vi "Bertta_v08_51.vi"() -> ()   [LabVIEW 2015]
panel:
  out "Started:":string
  in  "SHUTDOWN":bool
  in  "MASTER CONTROL":bool
  in  "Tab Control":T1(tab)
  in  "Read Seq":bool
  in  "Save Seq":bool
  in  "Configuration file":path=path "C:/Users/shresplab/Desktop/BerttaConfiguration.lvm" caption="Filename"
  in  "OK Button 2":bool
  out "Boolean":bool
  in  "User (initials)":string
  in  "Project name":string
  in  "Description":string
  out "Output file":string
  out "Sensor OK 6":bool
  out "Sensor OK 5":bool
  out "Sensor OK 4":bool
  out "Sensor OK 3":bool
  in  "OK Button":bool
  in  "Add comment":string
  out "PUMP 1":bool
  out "Target amount":dbl
  out "Scale weight":dbl
  out "Amount now":dbl
  out "Flow rate":dbl
  out "Time to target":dbl format="%<%H:%M:%S>t"
  out "Current step":dbl
  out "Target amount":dbl
  out "Amount now":dbl
  out "Tr":dbl
  out "Tj in":dbl
  out "Tj out":dbl
  out "T set":dbl
  out "Current step":i32
  out "RPM":dbl
  out "Torque 2":dbl
  out "Waveform Chart 5":dynamicdata(graph)
  out "Waveform Chart 6":dynamicdata(graph)
  out "Waveform Chart 7":dynamicdata(graph)
  out "Amount now":dbl
  out "Target amount":dbl
  out "Current step":dbl
  out "Time to target":dbl format="%<%H:%M:%S>t"
  out "Flow rate":dbl
  out "Amount now":dbl
  out "Scale weight":dbl
  out "Target amount":dbl
  out "PUMP 2":bool
  in  "Tab Control 2":T2(tab)
  out "Waveform Chart 3":dynamicdata(graph)
  out "Waveform Chart 8":dynamicdata(graph)
  out "Waveform Chart 11":dynamicdata(graph)
  out "Waveform Chart 9":dynamicdata(graph)
  out "Table":string[][](table)=[["14.8.2017 18.06.59", "0,000000", "417,670000", "-0,150000", "1,000000", "22,220000", "23,366837", "23,574959", "23,985852", "23,690000", "240,000000", "4,000000", "0,000000", "397,000000", "-397,000000", "1,000000"], ["14.8.2017 18.07.06", "0,000000", "417,640000", "-0,120000", "1,000000", "22,220000", "23,763115", "23,906257", "23,985694", "23,680000", "240,000000", "4,000000", "0,000000", "397,000000", "-397,000000", "1,000000"], ["14.8.2017 18.07.13", "0,000000", "417,640000", "-0,120000", "1,000000", "22,220000", "23,965922", "24,013440", "23,984906", "23,670000", "240,000000", "4,100000", "3,000000", "397,000000", "-397,000000", "1,000000"], ["14.8.2017 18.07.21", "0,000000", "417,640000", "-0,120000", "1,000000", "22,220000", "23,943860", "23,900110", "23,987113", "23,670000", "240,000000", "4,000000", "0,000000", "397,000000", "-397,000000", "1,000000"], ["14.8.2017 18.07.28", "0,000000", "417,640000", "-0,120000", "1,000000", "22,220000", "23,736328", "23,600018", "23,989004", "23,660000", "240,000000", "4,000000", "0,000000", "397,000000", "-397,000000", "1,000000"], ["14.8.2017 18.07.36", "0,000000", "417,640000", "-0,120000", "1,000000", "22,220000", "23,480910", "23,324538", "23,991053", "23,660000", "240,000000", "4,000000", "0,000000", "397,000000", "-397,000000", "1,000000"], ["14.8.2017 18.07.43", "0,000000", "417,640000", "-0,120000", "2,000000", "22,220000", "23,195579", "23,008270", "23,999093", "23,650000", "240,000000", "4,000000", "0,000000", "397,000000", "-397,000000", "1,000000"], ["14.8.2017 18.07.51", "0,000000", "417,650000", "-417,650000", "1,000000", "22,220000", "22,862541", "22,649021", "24,003979", "23,650000", "240,000000", "4,000000", "0,000000", "397,000000", "-397,000000", "2,000000"], ["14.8.2017 18.07.58", "0,000000", "417,640000", "0,010000", "1,000000", "22,220000", "22,541353", "22,354878", "24,005398", "23,650000", "240,000000", "4,000000", "0,000000", "397,000000", "-397,000000", "1,000000"], ["14.8.2017 18.08.06", "0,000000", "417,640000", "0,010000", "1,000000", "22,220000", "22,347931", "22,253738", "24,007605", "23,640000", "240,000000", "4,100000", "0,000000", "397,000000", "-397,000000", "1,000000"], ["14.8.2017 18.08.13", "0,000000", "417,640000", "0,010000", "1,000000", "22,220000", "22,329030", "22,302102", "24,006028", "23,640000", "240,000000", "4,000000", "0,000000", "395,820000", "-395,820000", "1,000000"], ["14.8.2017 18.08.20", "0,000000", "417,640000", "0,010000", "1,000000", "22,220000", "22,466849", "22,511320", "24,002403", "23,630000", "240,000000", "4,000000", "0,000000", "395,830000", "-0,010000", "1,000000"], ["14.8.2017 18.08.28", "0,000000", "417,640000", "0,010000", "1,000000", "22,220000", "22,707062", "22,835101", "24,000984", "23,620000", "240,000000", "4,000000", "0,000000", "395,830000", "-0,010000", "1,000000"], ["14.8.2017 18.08.35", "0,000000", "417,640000", "0,010000", "1,000000", "22,220000", "23,054104", "23,232979", "24,001299", "23,600000", "240,000000", "4,000000", "0,000000", "395,830000", "-0,010000", "1,000000"], ["14.8.2017 18.08.43", "0,000000", "417,640000", "0,010000", "1,000000", "22,220000", "23,412371", "23,522793", "24,002560", "23,590000", "240,000000", "4,000000", "0,000000", "395,820000", "0,000000", "1,000000"], ["14.8.2017 18.08.51", "0,000000", "417,640000", "0,010000", "1,000000", "22,220000", "23,596247", "23,656125", "24,003821", "23,580000", "240,000000", "4,000000", "0,000000", "395,820000", "0,000000", "1,000000"]]
  in  "T ext / T ext 2":enum32{"External 1", "External 2"}(radio)
  out "Sensor OK":bool
  in  "T fail":dbl=20.0
  out "Boolean 12":bool
  out "Boolean 7":bool
  out "Boolean 6":bool
  out "Boolean 5":bool
  out "Boolean 4":bool
  in  "?":bool
  in  "T setpoint":dbl=20.0
  in  "Lauda port":dbl=9.0
  out "Data out":dbl
  in  "Bypass select":enum32{"Tr", "Tj"}(radio)
  in  "TempSeq":dbl[][](array[numeric])=[[20.0, 45.0, 50.0, 46.0], [46.0, 50.0, 20.0, 51.0], [20.0, 50.0, 3.0, 25.0], [20.0, 20.0, 0.0, 20.0], [20.0, 20.0, 0.0, 20.0], [20.0, 20.0, 1000.0, 20.0]]
  out "T control":dbl
  out "Tr":dbl
  out "Tj in":dbl
  out "Tj out":dbl
  out "DT":dbl
  out "Elapsed":i32
  in  "PAUSE":bool
  out "Boolean 19":bool
  in  "Reset":bool
  in  "Treshold (Tset)":dbl=1.0
  in  "Tmax":dbl=199.0
  in  "Tmin":dbl=20.0
  out "Current step":i32
  out "Tset":dbl
  out "Waveform Chart":dynamicdata(graph)
  out "T external 2":dbl
  in  "Xe":dbl=1.0
  in  "Ring":u16(ring) items=["SCALE 1", "SCALE 2", "SCALE 3"]
  out "Data out":dbl
  out "Port":i32=10
  in  "Radio Buttons":enum32{"Reglo Digital", "Reglo Analog", "PAM"}(radio)=enum."Reglo Analog"
  out "Speed":dbl
  out "mA":dbl format="%#_2g"
  in  "Port":i32=16
  out "RPM":dbl format="%#_2g"
  out "Boolean 18":bool
  out "Boolean 17":bool
  out "Boolean 16":bool
  out "Boolean 15":bool
  out "Boolean 14":bool
  out "Boolean 13":bool
  out "Boolean 11":bool
  out "Boolean 10":bool
  out "Boolean 9":bool
  out "Boolean 8":bool
  in  "PumpSeq":dbl[][](array[numeric])=[[3.0, 3.0, 7.0], [2.0, 2.0, 2.0], [4.0, 2.0, 100.0], [0.0, 0.0, 0.0], [0.0, 0.0, 0.0], [0.0, 0.0, 0.0], [0.0, 0.0, 0.0], [0.0, 0.0, 0.0], [0.0, 0.0, 0.0], [0.0, 0.0, 0.0], [0.0, 1.0, 0.0]]
  in  "?":bool
  out "Flow rate (g/min)":dbl
  out "Time (min)":dbl
  out "Target (g)":dbl
  out "Scale reading":dbl
  out "Step amount now":dbl
  out "Time to target":dbl format="%<%H:%M:%S>t"
  in  "Grams / min":dbl
  out "Waveform Chart 2":dynamicdata(graph)
  in  "?":bool
  out "Total amount now":dbl
  out "Total time":dbl
  out "Total amount target":dbl
  out "Boolean 20":bool
  in  "Reset 2":bool
  out "Waveform Chart 10":dynamicdata(graph)
  in  "Reset 3":bool
  out "Boolean 31":bool
  out "Total amount target 2":dbl
  out "Total time 2":dbl
  out "Boolean 30":bool
  out "Boolean 29":bool
  out "Boolean 28":bool
  out "Boolean 27":bool
  out "Boolean 26":bool
  out "Boolean 25":bool
  out "Boolean 24":bool
  out "Boolean 23":bool
  out "Boolean 22":bool
  out "Boolean 21":bool
  in  "PumpSeq 2":dbl[][](array[numeric])=[[3.0, 3.0, 7.0], [2.0, 2.0, 2.0], [4.0, 2.0, 100.0], [0.0, 0.0, 0.0], [0.0, 0.0, 0.0], [0.0, 0.0, 0.0], [0.0, 0.0, 0.0], [0.0, 0.0, 0.0], [0.0, 0.0, 0.0], [0.0, 0.0, 0.0], [0.0, 1.0, 0.0]]
  in  "Ring 2":u16(ring)=1 items=["SCALE 1", "SCALE 2", "SCALE 3"]
  out "Data out 2":dbl
  out "Port 3":i32=10
  in  "Radio Buttons 2":enum32{"Reglo Digital", "Reglo Analog", "PAM"}(radio)
  out "RPM":dbl format="%#_2g"
  in  "Port":i32=15
  out "mA":dbl format="%#_2g"
  out "Speed":dbl
  in  "?":bool
  in  "Grams / min":dbl
  out "Time (min)":dbl
  out "Target (g)":dbl
  out "Total amount now":dbl
  out "Time to target":dbl format="%<%H:%M:%S>t"
  in  "?":bool
  out "Step amount now":dbl
  out "Scale reading":dbl
  out "Flow rate (g/min)":dbl
  in  "Bypass select 2":enum32{"Remote", "Manual"}(radio)
  in  "Port":dbl=13.0
  out "RPM":dbl
  out "Torque":dbl
  in  "Set RPM":dbl(slide) scale=0.0..500.0
  out "Waveform Chart 4":dynamicdata(graph)
  out "DAQ 9217 (PT100)":errorcluster
  # "PUMP & SCALE 1"
  # "PUMP & SCALE 2"
  # "STEP"
  # "STEP"
  # "TOTAL"
  # "TOTAL"
  # "Temperature sensor:"
  # "Manual control:"
  # "Tinit     >    Tset       Min. time      Tfail"
  # "Manual control / end of sequence"
  # "Manual control"
  # "Secondary temperature sensor"
  # "Device communication"
  # "Grams    /   min"
  # "End of sequence"
  # "Manual control"
  # "Device communication"
  # "Pump configuration"
  # "Scale configuration"
  # "Grams    /   min"
  # "End of sequence"
  # "Manual control"
  # "Device communication"
  # "Pump configuration"
  # "Scale configuration"
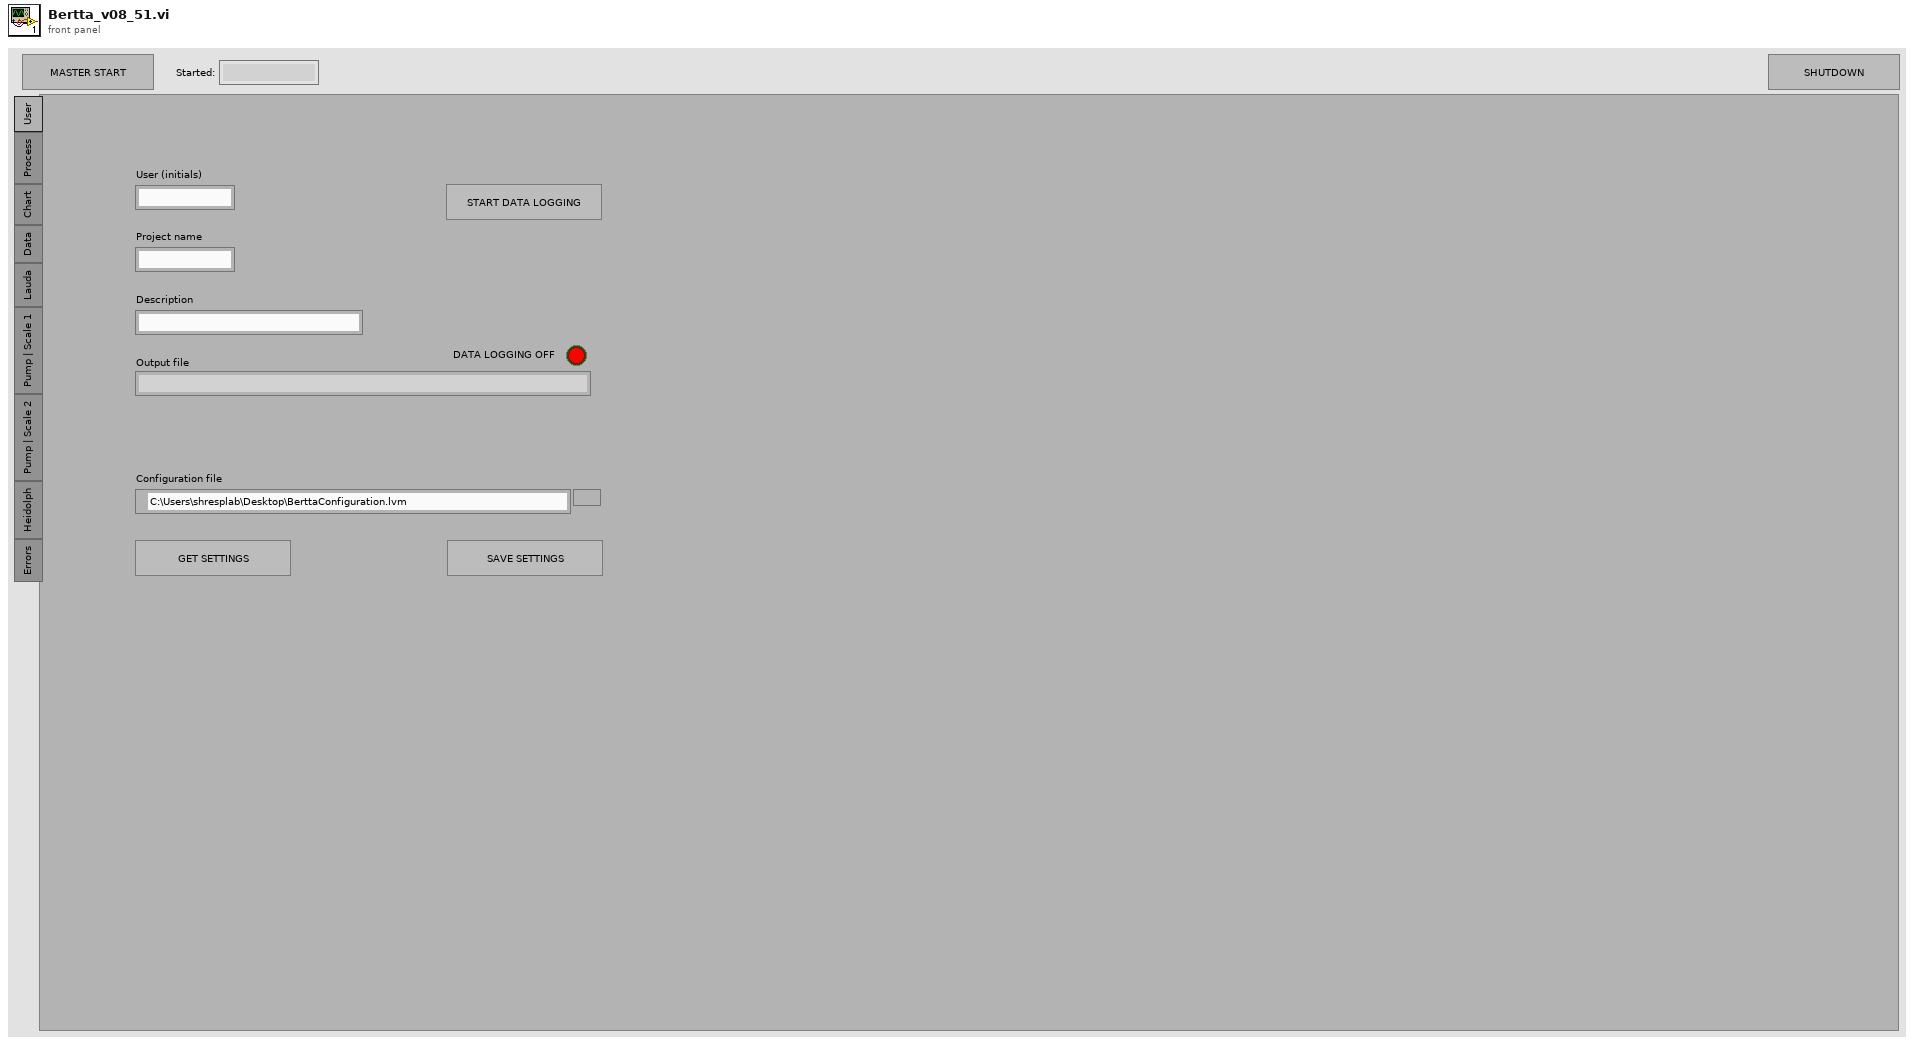
[diagram p1: front panel]
types:
  T1 = enum32{"User", "Process", "Chart", "Data", "Lauda", "Pump | Scale 1", "Pump | Scale 2", "Heidolph", "Errors"}
  T2 = enum32{"Temperatures", "Scale / Pump 1", "Scale / Pump 2", "RPM / torque"}
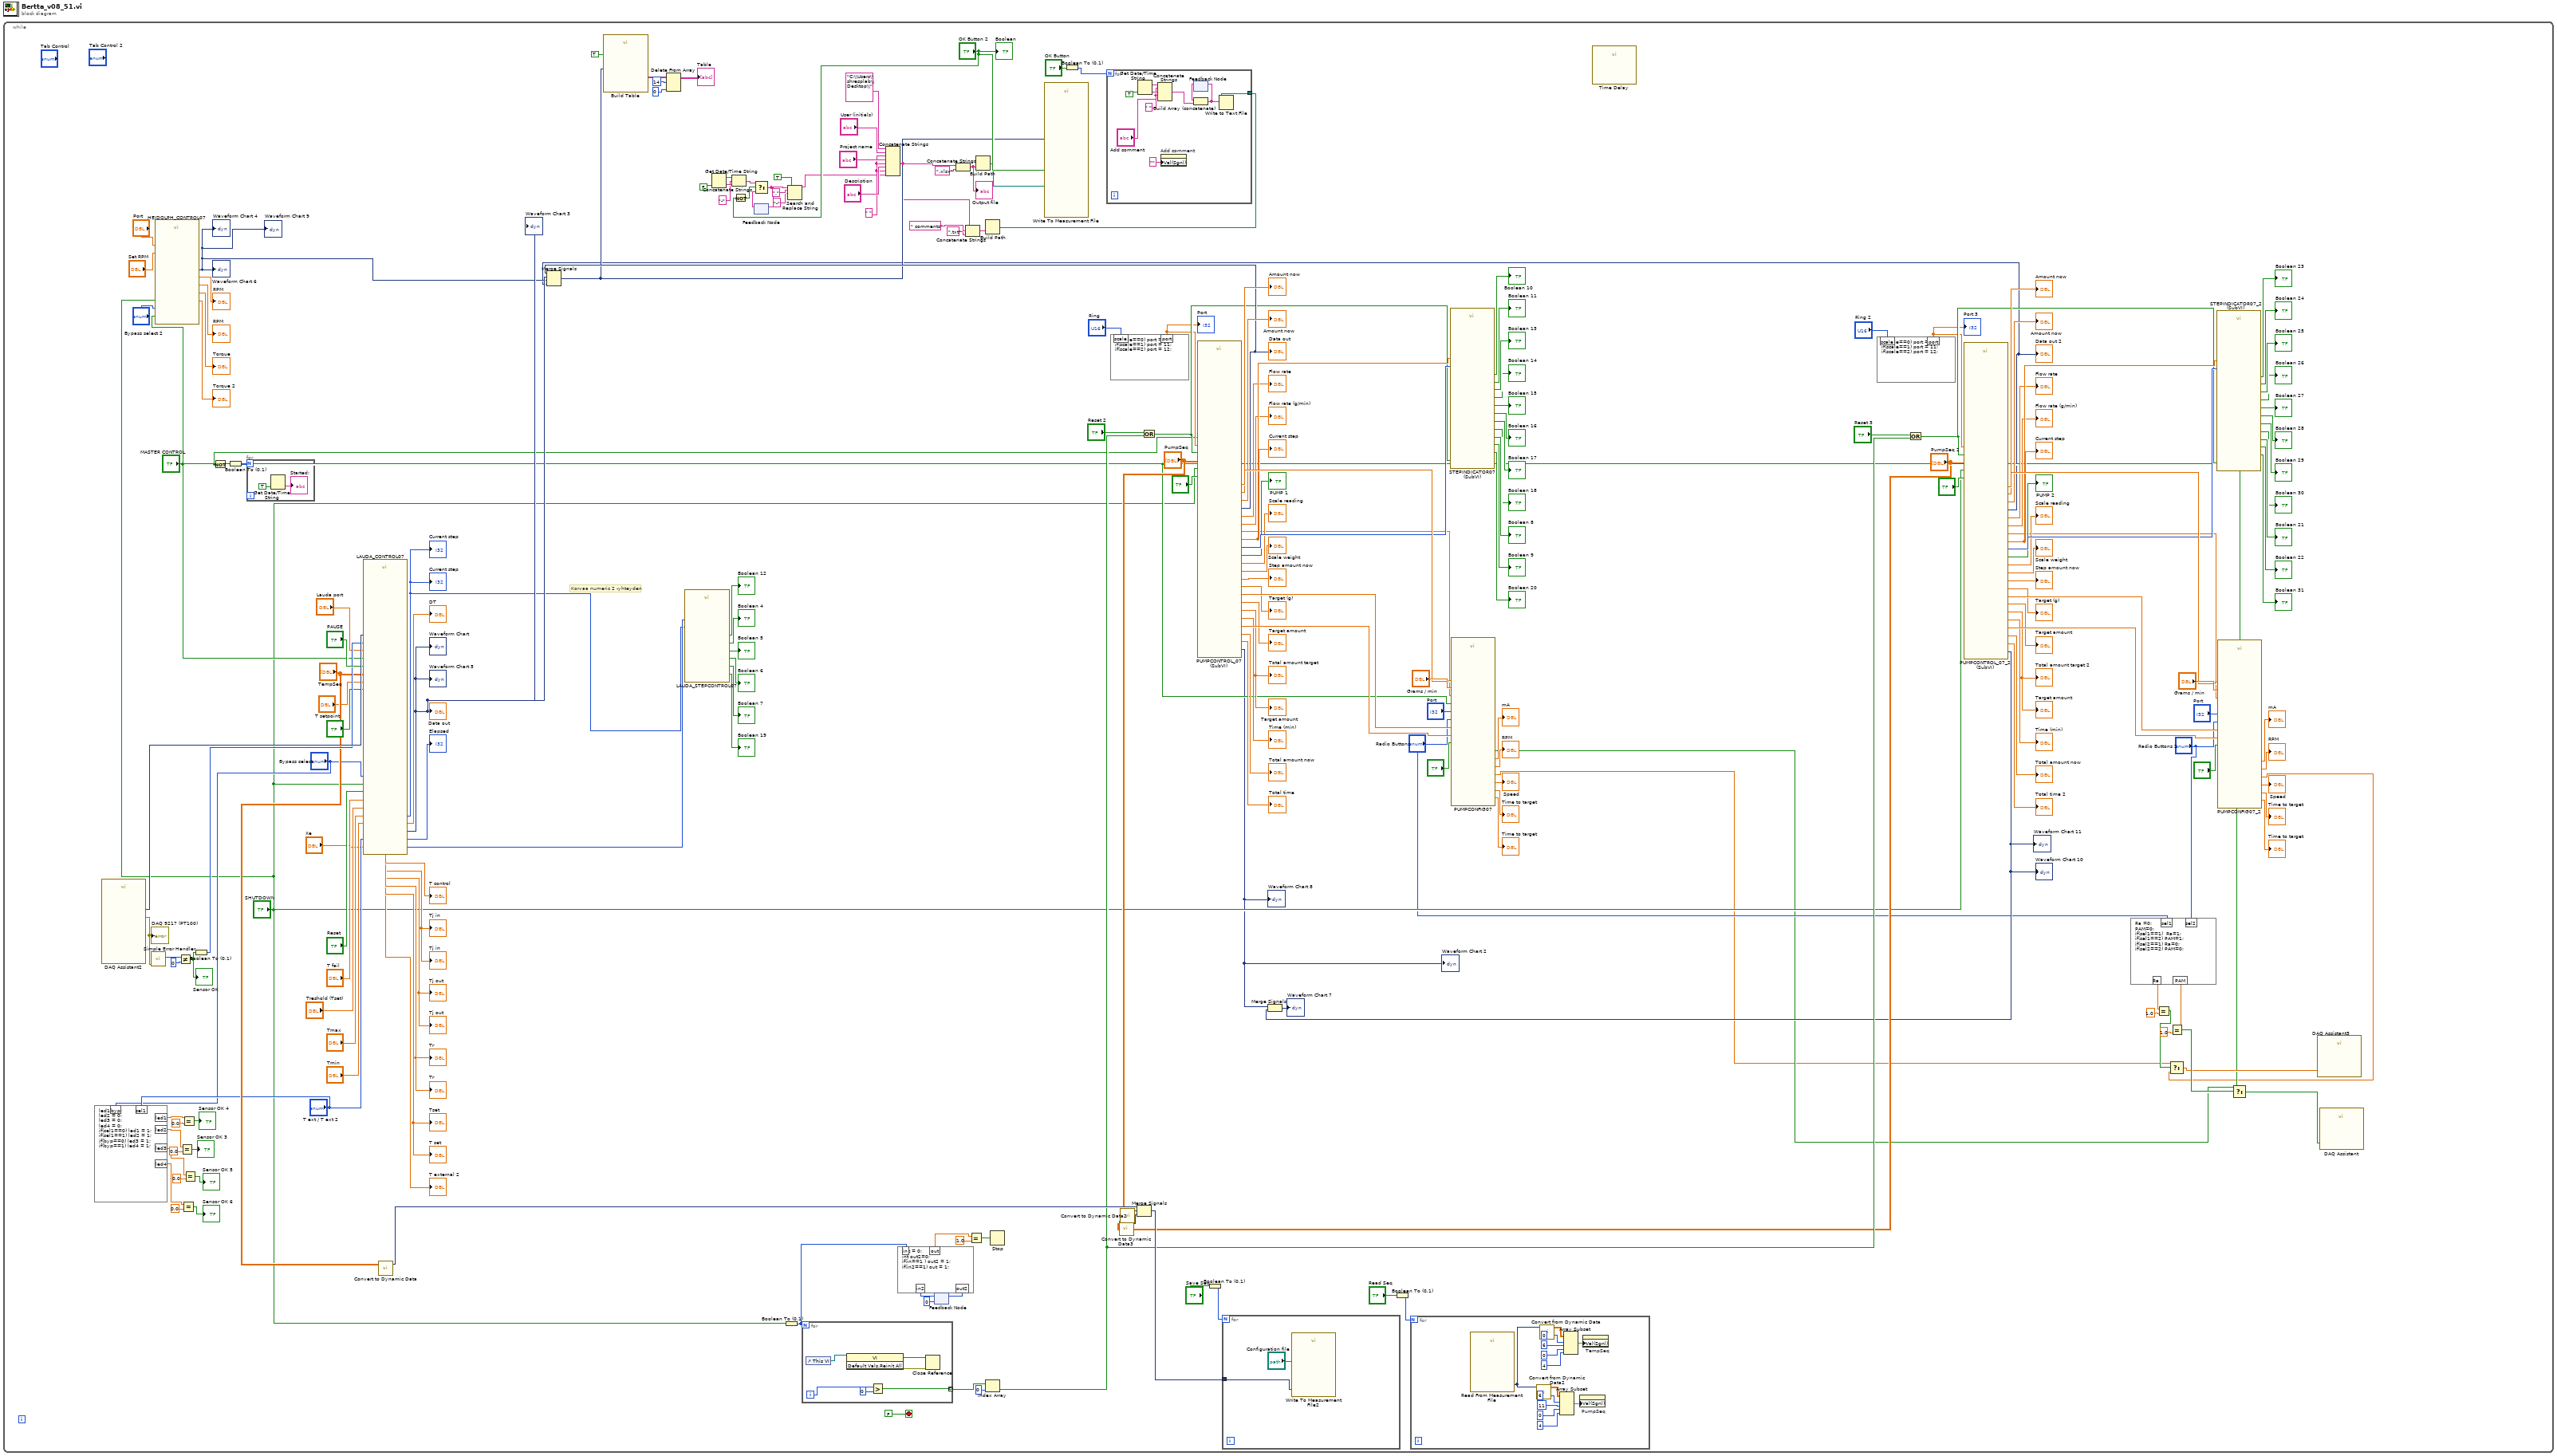
[diagram p0: block diagram]
diagram:
  n1 = while {
    stop <- FALSE stop-if-true
    w157 = " "
    # "Korvaa numeric 2 -yhteyden"
    n2 = formula code="led1 = 0;\nled2 = 0;\nled3 = 0;\nled4 = 0;\nif(sel1==0) led1 = 1;\nif(sel1==1) led2 = 1;\nif(byp==0) led3 = 1;\nif(byp==1) led4 = 1;"("sel1"="T ext / T ext 2", "byp"="Bypass select") -> ("led1"=w81:dbl, "led2"=w79:dbl, "led3"=w74:dbl, "led4"=w73:dbl)
    n3 = call "DAQ Assistant2"() -> ("data"=w220:dynamicdata, "error out"=w164:errorcluster)  [unwired: 17 in, 1 out]
    "DAQ 9217 (PT100)" <- w164
    n4 = call <vilib>:"Simple Error Handler.vi"("error in (no error)"=w164) -> ("code out"=w163:i32)  [unwired: 4 in, 4 out]
    n5 = call "HEIDOLPH_CONTROL07.vi"("master"="MASTER CONTROL", "shutdown"="SHUTDOWN", "Bypass select"="Bypass select 2", "Set RPM"="Set RPM", "Device port"="Port") -> ("Dynamic Data"=w169:dynamicdata, "RPM"=→"RPM":dbl, "RPM 2"=→"RPM":dbl, "Torque"=→"Torque":dbl, "Torque 2"=→"Torque 2":dbl)  [unwired: 2 in]
    "Waveform Chart 4" <- w169
    "Waveform Chart 6" <- w169
    "Waveform Chart 9" <- w169
    n6 = Not Equal?(x=w163, y=0) -> (x != y?=w129:bool)
    "Sensor OK" <- w129
    n7 = Equal?(x=w79, y=0.0) -> (x = y?=→"Sensor OK 3":bool)
    n8 = Equal?(x=w73, y=0.0) -> (x = y?=→"Sensor OK 6":bool)
    n9 = Equal?(x=w81, y=0.0) -> (x = y?=→"Sensor OK 4":bool)
    n10 = Equal?(x=w74, y=0.0) -> (x = y?=→"Sensor OK 5":bool)
    n11 = Boolean To (0,1)(Boolean=w129) -> (0, 1=w161:i16)
    n12 = Not(x="MASTER CONTROL") -> (.not. x?=w146:bool)
    n13 = Boolean To (0,1)(Boolean=w146) -> (0, 1=w147:i16)
    n14 = for {
      N: w147 -> [_]
      n15 = Get Date/Time String(want seconds? (F)=TRUE) -> (time string=→"Started:":string)  [unwired: 2 in, 1 out]
    }
    n16 = call "LAUDA_CONTROL07.vi"("Bypass"="?", "PAUSE"="PAUSE", "data"=w220, "Seq"="TempSeq", "Lauda port"="Lauda port", "Tbypass"="T setpoint", "Treshold"="Treshold (Tset)", "Bypass select"="Bypass select", "err"=w161, "Shutdown"="SHUTDOWN", "Master Start"="MASTER CONTROL", "Reset"="Reset", "Tfail (manual)"="T fail", "Tmax"="Tmax", "Xe"="Xe", "T ext / T ext 2"="T ext / T ext 2", "Tmin"="Tmin") -> ("Tj in"=→"Tj in" →"Tj in":dbl, "DT"=→"DT":dbl, "Tj out"=→"Tj out" →"Tj out":dbl, "Tset"=→"Tset" →"T set":dbl, "Dynamic Data"=w171:dynamicdata, "T ext 2"=→"T external 2":dbl, "Numeric"=w150:i16, "T control"=→"T control":dbl, "Current step"=w2:i32, "Elapsed"=→"Elapsed":i32, "Tr"=→"Tr" →"Tr":dbl)
    "Waveform Chart 3" <- w171
    "Waveform Chart" <- w171
    "Current step" <- w2
    "Data out" <- w171
    "Waveform Chart 5" <- w171
    "Current step" <- w2
    n17 = call "Convert to Dynamic Data"("2D Array"="TempSeq") -> ("Dynamic Data Type"=w139:dynamicdata)  [unwired: 3 in]
    n18 = call "LAUDA_STEPCONTROL07.vi"("Numeric 2"=w2, "Numeric"=w150) -> ("Boolean 13"=→"Boolean 19":bool, "Boolean 6"=→"Boolean 6":bool, "Boolean 5"=→"Boolean 5":bool, "Boolean 4"=→"Boolean 4":bool, "Boolean 7"=→"Boolean 7":bool, "Boolean 12"=→"Boolean 12":bool)  [unwired: 4 in]
    n19 = Get Date/Time String(want seconds? (F)=FALSE) -> (date string=w117:string, time string=w112:string)  [unwired: 2 in]
    n20 = Concatenate Strings(w117, "-" ("string"), w112) -> (w116:string)
    n21 = Not(x="OK Button 2") -> (.not. x?=w113:bool)
    n22 = feedback #1() -> (w115:string)  [unwired: 1 in]
    n23 = Select(t=w116, s=w113, f=w115) -> (s? t:f=w108:string)
    n24 = feedback-in #1(w108) -> ()
    n25 = Boolean To (0,1)(Boolean="SHUTDOWN") -> (0, 1=w87:i16)
    n26 = Search and Replace String(replace all?=TRUE ("replace all? (F)"), input string=w108, search string=".", replace string="-" ("replace string (\"\")")) -> (result string=w107:string)  [unwired: 4 in, 3 out]
    n27 = for {
      N: w87 -> [_]
      tunnel: [w248] -> w142 mode=indexing
      i -> [w250]
      n28 = control-ref of="This VI"() -> (w253:refnum<vi>)
      n29 = invoke class="VI" method="Default Vals.Reinit All"(reference=w253) -> (reference out=w251:refnum<vi>, error out=w252:errorcluster)  [unwired: 2 in, 1 out]
      n30 = Greater?(x=w250, y=0) -> (0:w248:bool)
      n31 = Close Reference(reference=w251, error in (no error)=w252) -> ()  [unwired: 1 out]
    }
    n32 = Concatenate Strings("C:\\Users\\shresplab\\Desktop\\", "User (initials)", w157, "Project name", w157, "Description", w157, w107) -> (w97:string)
    n33 = feedback #2(0) -> (w85:i32)
    n34 = formula code="out = 0;\nint out2=0;\nif(in==1 ) out2 = 1;\nif(in2==1) out = 1;"("in"=w87, "in2"=w85) -> ("out"=w89:dbl, "out2"=w86:i32)
    n35 = feedback-in #2(w86) -> ()
    n36 = Concatenate Strings(w97, ".xlsx") -> (w100:string)
    "Output file" <- w100
    n37 = Concatenate Strings(w97, " comments" ("string"), ".txt" ("string")) -> (w94:string)
    n38 = Equal?(x=w89, y=1.0) -> (x = y?=w88:bool)
    n39 = Build Path(name or relative path=w100) -> (appended path=w98:path)  [unwired: 1 in]
    n40 = Index Array(array=w142, index=0) -> (element=w25:bool)
    n41 = Build Path(name or relative path=w94) -> (appended path=w93:path)  [unwired: 1 in]
    n42 = Stop(stop? (T)=w88) -> ()
    n43 = Boolean To (0,1)(Boolean="OK Button") -> (0, 1=w92:i16)
    n44 = for {
      N: w92 -> [_]
      tunnel: w93 -> [w225]
      w229 = " " ("string")
      n45 = Get Date/Time String(want seconds? (F)=TRUE) -> (date string=w232:string, time string=w230:string)  [unwired: 2 in]
      n46 = Concatenate Strings(w232, w229, w230, w229, "Add comment") -> (w228:string)
      n47 = property on="Add comment" class="Str"("Val(Sgnl)"="" ("Value (Signaling)")) -> ()  [unwired: 2 in, 2 out]
      n48 = feedback #3() -> (w227:string[])  [unwired: 1 in]
      n49 = Build Array (concatenate)(w227, w228) -> (w226:string[])
      n50 = feedback-in #3(w226) -> ()
      n51 = Write to Text File(file (use dialog)=w225, text=w226) -> ()  [unwired: 2 in, 3 out]
    }
    n52 = formula code="if(scale==0) port = 10;\nif(scale==1) port = 11;\nif(scale==2) port = 12;"("scale"="Ring") -> ("port"=w119:dbl)
    "Port" <- w119
    n53 = call "Convert to Dynamic Data3"("2D Array"="PumpSeq 2") -> ("Dynamic Data Type"=w23:dynamicdata)  [unwired: 3 in]
    n54 = call "Convert to Dynamic Data2"("2D Array"="PumpSeq") -> ("Dynamic Data Type"=w137:dynamicdata)  [unwired: 3 in]
    n55 = Merge Signals(w139, w137, w23) -> (w136:dynamicdata)
    n56 = Or(x="Reset 2", y=w25) -> (x .or. y?=w128:bool)
    n57 = call "PUMPCONTROL_07 (SubVI).vi"("Port"=w119, "Pause"="MASTER CONTROL", "Master start"="?", "shutdown"="SHUTDOWN", "Seq in"="PumpSeq", "reset"=w128) -> ("Amount now"=→"Amount now":dbl, "Amount now 2"=→"Amount now":dbl, "Flow rate out"=w152:dbl, "Step amount now"=→"Step amount now":dbl, "Total amount now"=→"Total amount now":dbl, "Total time"=→"Total time":dbl, "Numeric 2"=w216:i16, "PUMP 1"=→"PUMP 1":bool, "Numeric"=w212:dbl, "Flow rate"=→"Flow rate":dbl, "Dynamic Data"=w170:dynamicdata, "Target amount"=→"Target amount":dbl, "Time (min) 2"=w217:dbl, "Target amount 2"=→"Total amount target" →"Target amount":dbl, "Scale reading"=→"Scale reading":dbl, "Flow rate (g/min)"=→"Flow rate (g/min)":dbl, "Target (g) 2"=w218:dbl, "Target (g)"=→"Target (g)":dbl, "Time (min)"=→"Time (min)":dbl, "Waveform Chart 2"=w5:dynamicdata, "Scale weight"=→"Scale weight":dbl, "Amount (g)"=w219:dbl)
    "Waveform Chart 2" <- w5
    "Current step" <- w212
    "Data out" <- w170
    "Waveform Chart 8" <- w5
    n58 = Boolean To (0,1)(Boolean="Save Seq") -> (0, 1=w135:i16)
    n59 = for {
      N: w135 -> [_]
      tunnel: w136 -> [w247]
      n60 = call "Write To Measurement File2"("Signals"=w247, "Filename"="Configuration file") -> ()  [unwired: 15 in, 3 out]
    }
    n61 = Boolean To (0,1)(Boolean="Read Seq") -> (0, 1=w132:i16)
    n62 = for {
      N: w132 -> [_]
      n63 = call "Read From Measurement File"() -> ("Signals"=w235:dynamicdata)  [unwired: 6 in, 5 out]
      n64 = call "Convert from Dynamic Data2"("Dynamic Data Type"=w235) -> ("Array"=w234:dbl[][])  [unwired: 3 in]
      n65 = call "Convert from Dynamic Data"("Dynamic Data Type"=w235) -> ("Array"=w243:dbl[][])  [unwired: 3 in]
      n66 = Array Subset(array=w234, index (row)=6 ("index"), length (row)=11 ("length"), index (col)=0 ("index"), length (col)=4 ("length")) -> (w233:dbl[][])
      n67 = Array Subset(array=w243, index (row)=0 ("index"), length (row)=6 ("length"), index (col)=0 ("index"), length (col)=4 ("length")) -> (w240:dbl[][])
      n68 = property on="PumpSeq" class="Arr (strict)"("Val(Sgnl)"=w233) -> ()  [unwired: 2 in, 2 out]
      n69 = property on="TempSeq" class="Arr (strict)"("Val(Sgnl)"=w240) -> ()  [unwired: 2 in, 2 out]
    }
    n70 = call "STEPINDICATOR07 (SubVI).vi"("Numeric"=w212, "Numeric 2"=w216, "Reset"=w128) -> ("Boolean 18"=→"Boolean 18":bool, "Boolean 8"=→"Boolean 8":bool, "Boolean 9"=→"Boolean 9":bool, "Boolean 17"=→"Boolean 17":bool, "Boolean 10"=→"Boolean 10":bool, "Boolean 16"=→"Boolean 16":bool, "Boolean 11"=→"Boolean 11":bool, "Boolean 15"=→"Boolean 15":bool, "Boolean 14"=→"Boolean 14":bool, "Boolean 13"=→"Boolean 13":bool, "Boolean 19"=→"Boolean 20":bool)  [unwired: 2 in]
    n71 = call "PUMPCONFIG07.vi"(0:"?", "Radio Buttons"="Radio Buttons", "Bypass (g/min)"="Grams / min", "Target (g) in"=w218, "Amount (g)"=w219, "Time (min) in"=w217, "Flow rate in"=w152, "OK Button"="MASTER CONTROL", "Port"="Port") -> ("Time to target 2"=→"Time to target":dbl, "Time to target"=→"Time to target":dbl, "mA"=→"mA":dbl, "signal"=w9:dbl, "Speed"=→"Speed":dbl, "RPM"=→"RPM":dbl, "Array"=w11:bool[])
    n72 = call "Time Delay"() -> ()  [unwired: 11 in, 1 out]
    n73 = formula code="if(scale==0) port = 10;\nif(scale==1) port = 11;\nif(scale==2) port = 12;"("scale"="Ring 2") -> ("port"=w26:dbl)
    "Port 3" <- w26
    n74 = Or(x="Reset 3", y=w25) -> (x .or. y?=w29:bool)
    n75 = call "PUMPCONTROL_07_2 (SubVI).vi"("Port"=w26, "Pause"="MASTER CONTROL", "Master start"="?", "shutdown"="SHUTDOWN", "Seq in"="PumpSeq 2", "reset"=w29) -> ("Amount now"=→"Amount now":dbl, "Amount now 2"=→"Amount now":dbl, "Flow rate out"=w33:dbl, "Step amount now"=→"Step amount now":dbl, "Total amount now"=→"Total amount now":dbl, "Total time"=→"Total time 2":dbl, "Numeric 2"=w65:i16, "PUMP 1"=→"PUMP 2":bool, "Numeric"=w62:dbl, "Flow rate"=→"Flow rate":dbl, "Dynamic Data"=w3:dynamicdata, "Target amount"=→"Target amount":dbl, "Time (min) 2"=w66:dbl, "Target amount 2"=→"Total amount target 2" →"Target amount":dbl, "Scale reading"=→"Scale reading":dbl, "Flow rate (g/min)"=→"Flow rate (g/min)":dbl, "Target (g) 2"=w67:dbl, "Target (g)"=→"Target (g)":dbl, "Time (min)"=→"Time (min)":dbl, "Waveform Chart 2"=w20:dynamicdata, "Scale weight"=→"Scale weight":dbl, "Amount (g)"=w68:dbl)
    "Waveform Chart 10" <- w20
    "Current step" <- w62
    "Data out 2" <- w3
    "Waveform Chart 11" <- w20
    n76 = Merge Signals(w170, w171, w169, w3) -> (w104:dynamicdata)
    n77 = call "Build Table"("Include time data"=TRUE, "Signals"=w104) -> ("Table"=w103:string[][])  [unwired: 3 in, 6 out]
    n78 = Delete From Array(array=w103, length=14, index (col)=0 ("index (row)")) -> (array with subset deleted=→"Table":string[][])  [unwired: 1 in, 1 out]
    n79 = call "Write To Measurement File"("Signals"=w104, "Enable"="OK Button 2", "Filename"=w98) -> ()  [unwired: 14 in, 3 out]
    n80 = Merge Signals(w5, w20) -> (→"Waveform Chart 7":dynamicdata)
    n81 = formula code="Ra =0;\nPAM=0;\nif(sel1==1)  Ra=1;\nif(sel1==2) PAM=1;\nif(sel2==1) Ra=0;\nif(sel2==2) PAM=0;"("sel1"="Radio Buttons", "sel2"="Radio Buttons 2") -> ("Ra"=w17:dbl, "PAM"=w14:dbl)
    n82 = Equal?(x=w17, y=1.0) -> (x = y?=w13:bool)
    n83 = Equal?(x=w14, y=1.0) -> (x = y?=w12:bool)
    n84 = call "STEPINDICATOR07_2 (SubVI).vi"("Numeric"=w62, "Numeric 2"=w65, "Reset"=w29) -> ("Boolean 18"=→"Boolean 30":bool, "Boolean 8"=→"Boolean 21":bool, "Boolean 9"=→"Boolean 22":bool, "Boolean 17"=→"Boolean 29":bool, "Boolean 10"=→"Boolean 23":bool, "Boolean 16"=→"Boolean 28":bool, "Boolean 11"=→"Boolean 24":bool, "Boolean 15"=→"Boolean 27":bool, "Boolean 14"=→"Boolean 26":bool, "Boolean 13"=→"Boolean 25":bool, "Boolean 19"=→"Boolean 31":bool)  [unwired: 2 in]
    n85 = call "PUMPCONFIG07_2.vi"(0:"?", "Radio Buttons"="Radio Buttons 2", "Bypass (g/min)"="Grams / min", "Target (g) in"=w67, "Amount (g)"=w68, "Time (min) in"=w66, "Flow rate in"=w33, "OK Button"="MASTER CONTROL", "Port"="Port") -> ("Time to target 2"=→"Time to target":dbl, "Time to target"=→"Time to target":dbl, "mA"=→"mA":dbl, "signal"=w6:dbl, "Speed"=→"Speed":dbl, "RPM"=→"RPM":dbl, "Array"=w7:bool[])
    n86 = Select(t=w9, s=w13, f=w6) -> (s? t:f=w8:dbl)
    n87 = Select(t=w11, s=w12, f=w7) -> (s? t:f=w10:bool[])
    n88 = call "DAQ Assistant3"("data"=w8) -> ()  [unwired: 17 in, 2 out]
    n89 = call "DAQ Assistant"("data"=w10) -> ()  [unwired: 17 in, 2 out]
    "Boolean" <- "OK Button 2"
  }
